vi "Plot Helper (Vector).vi"(8 "error in (no error)":errorcluster, 9 "y vector":dbl[](array[numeric]), 10 "x vector":dbl[](array[numeric]), 11 "2D Plot Class Obj Array in":refnum<class "2D Plot Datatype.lvclass">[](array[class])) -> (0 "error out":errorcluster, 3 "2D Plot Class Obj Array out":refnum<class "2D Plot Datatype.lvclass">[](array[class]))   [LabVIEW 2020, in "2D Feather Datatype.lvclass"]
doc: "Graphs vectors that emanate from equally spaced points along a horizontal axis at zero. Multiple references to this VI generate multiple plots on the same graph."
uses:
  <vilib>/Math Plots/2D Math Plots/2D Feather/2D Feather Datatype/2D Feather Datatype.lvclass
  <vilib>/Math Plots/2D Math Plots/2D Plot/2D Plot Datatype/2D Plot Datatype.lvclass
  e:/builds/penguin/labview/branches/2020/dev/dist/vi.lib/Math Plots/2D Math Plots/2D Plot/2D Plot Datatype/2D Plot Datatype.lvclass
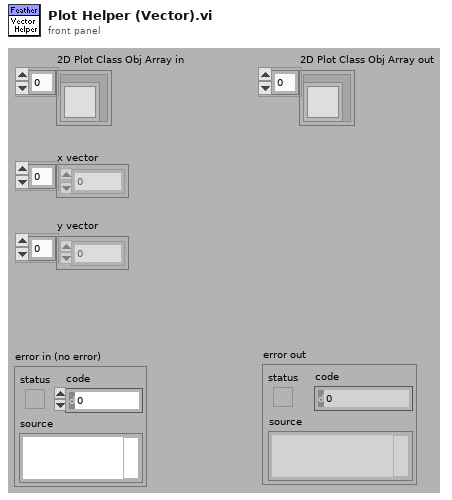
[diagram p1: front panel]
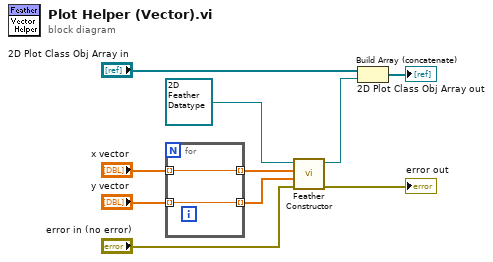
[diagram p0: block diagram]
diagram:
  n1 = for {
    tunnel: [w12] -> w4 mode=indexing
    tunnel: "x vector" -> [w12] mode=indexing
    tunnel: [w11] -> w2 mode=indexing
    tunnel: "y vector" -> [w11] mode=indexing
  }
  n2 = call <vilib>:"Feather Constructor.vi"("error in (no error)"="error in (no error)", "y vector"=w2, "x vector"=w4, "2D Feather Datatype.lvclass in"=refnum<class "2D Feather Datatype.lvclass"> refnum ("3D Quiver Datatype.lvclass in")) -> ("error out"=→"error out":errorcluster, "2D Feather Datatype.lvclass out"=w6:refnum<class "2D Feather Datatype.lvclass">)  [unwired: 1 in, 5 out]
  n3 = Build Array (concatenate)("2D Plot Class Obj Array in", w6) -> (→"2D Plot Class Obj Array out":refnum<class "2D Plot Datatype.lvclass">[])
